vi "Save Config.vi"(4 "Error In":errorcluster, 5 "Configuration In":T1, 7 "File Path In":path) -> (0 "Error Out":errorcluster, 1 "Configration Out":T1, 2 "Cancelled":bool, 3 "File Path Out":path)   [LabVIEW 2018]
uses:
  Type Defs/Configration.ctl
  GC-MSMSDevlopment/Type/_RT Configuration 2.ctl
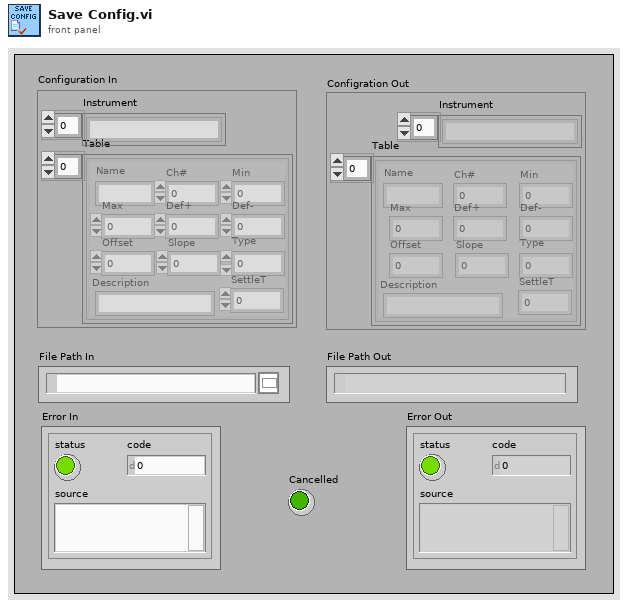
[diagram p1: front panel]
types:
  T1 = typedef "Configration.ctl" = cluster{"Table":T2[], "Instrument":string[]}
  T2 = typedef "_RT Configuration 2.ctl" = cluster{"Name":string, "Ch#":u8, "Min":dbl, "Max":dbl, "Def+":dbl, "Def-":dbl, "Offset":dbl, "Slope":dbl, "Type":u8, "Description":string, "SettleT":dbl}
  T3 = enum16{"open", "replace", "create", "open or create", "replace or create", "replace or create with confirmation"}
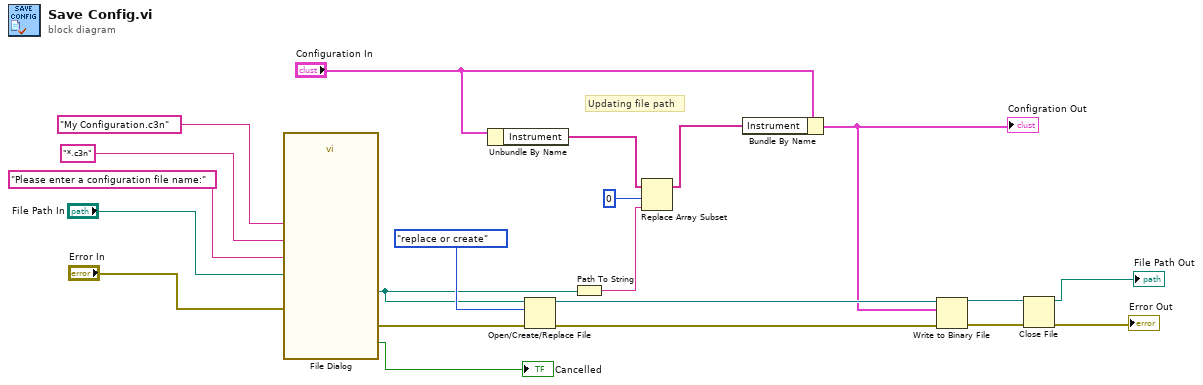
[diagram p0: block diagram]
diagram:
  # "Updating file path"
  n1 = call "File Dialog"("start path"="File Path In", "prompt"="Please enter a configuration file name:", "default name"="My Configuration.c3n" ("pattern (*.cfg)"), "error in"="Error In", "pattern (all files)"="*.c3n" ("pattern (*.cfg)")) -> ("selected path"=w10:path, "cancelled"=→"Cancelled":bool, "error out"=w16:errorcluster)  [unwired: 7 in, 1 out]
  n2 = Unbundle By Name("Configuration In") -> ("Instrument"=w12:string[])
  n3 = Open/Create/Replace File(file path (use dialog)=w10, error in=w16, operation (0:open)=T3."replace or create") -> (refnum out=w8:refnum<file>, error out=w7:errorcluster)  [unwired: 3 in, 1 out]
  n4 = Path To String(path=w10) -> (string=w9:string)
  n5 = Replace Array Subset(array=w12, new element=w9, index=0) -> (w14:string[])
  n6 = Bundle By Name(cluster="Configuration In", "Instrument"=w14) -> (w6:T1)
  "Configration Out" <- w6
  n7 = Write to Binary File(file (use dialog)=w8, data=w6, error in=w7) -> (refnum out=w4:refnum<file>, error out=w5:errorcluster)  [unwired: 3 in, 1 out]
  n8 = Close File(refnum=w4, error in=w5) -> (path=→"File Path Out":path, error out=→"Error Out":errorcluster)
